vi "Write Config Ref.vi"(8 "error in (no error)":errorcluster, 10 "Config File Refnum":variant, 11 "Base In":refnum<class "Base.lvclass">) -> (0 "error out":errorcluster, 3 "Base Out":refnum<class "Base.lvclass">)   [LabVIEW 2020, in "Base.lvclass"]
doc: "For the configuration interface to work, the class implementing the interface needs to save the reference to the file in the class attributes. This is an accessor for that attribute which must be implemented by the class."
uses:
  Base.lvclass
  Base.lvclass/Base.ctl
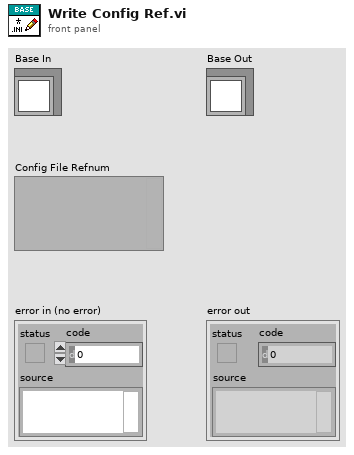
[diagram p1: front panel]
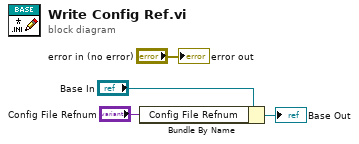
[diagram p0: block diagram]
diagram:
  n1 = Bundle By Name(cluster="Base In", "Config File Refnum"="Config File Refnum") -> (→"Base Out":refnum<class "Base.lvclass">)
  "error out" <- "error in (no error)"
